vi "PrototypeV2_control.vi"() -> ()   [LabVIEW 2019]
uses:
  0f690846-c94a-4028-9fe1-d10e28cf598c.vi
  <vilib>/Instr/_visa.llb/VISA Configure Serial Port (Instr).vi
panel:
  out "elapsed time":dbl
  in  "SAS file":path
  in  "SAS VISA":refnum<visa-resource-name>
  out "CONV2":cluster{dbl, dbl, dbl}(graph)
  out "converter2 file":path
  out "controller file":path
  out "converter1 file":path
  in  "CONVERTER 2 PORT":refnum<visa-resource-name>="COM5"
  out "sync":bool
  in  "CONVERTER 1 PORT":refnum<visa-resource-name>="COM4"
  out "sync":bool
  out "CONV1":cluster{dbl, dbl, dbl}(graph)
  out "3.3V REG":cluster{dbl, dbl}(graph)
  out "5V REG":cluster{dbl, dbl}(graph)
  out "BUS":cluster{dbl, dbl, dbl}(graph)
  in  "project name":string
  in  "START":bool
  in  "CONTROLLER PORT":refnum<visa-resource-name>="COM3"
  out "sync":bool
  in  "STOP":bool
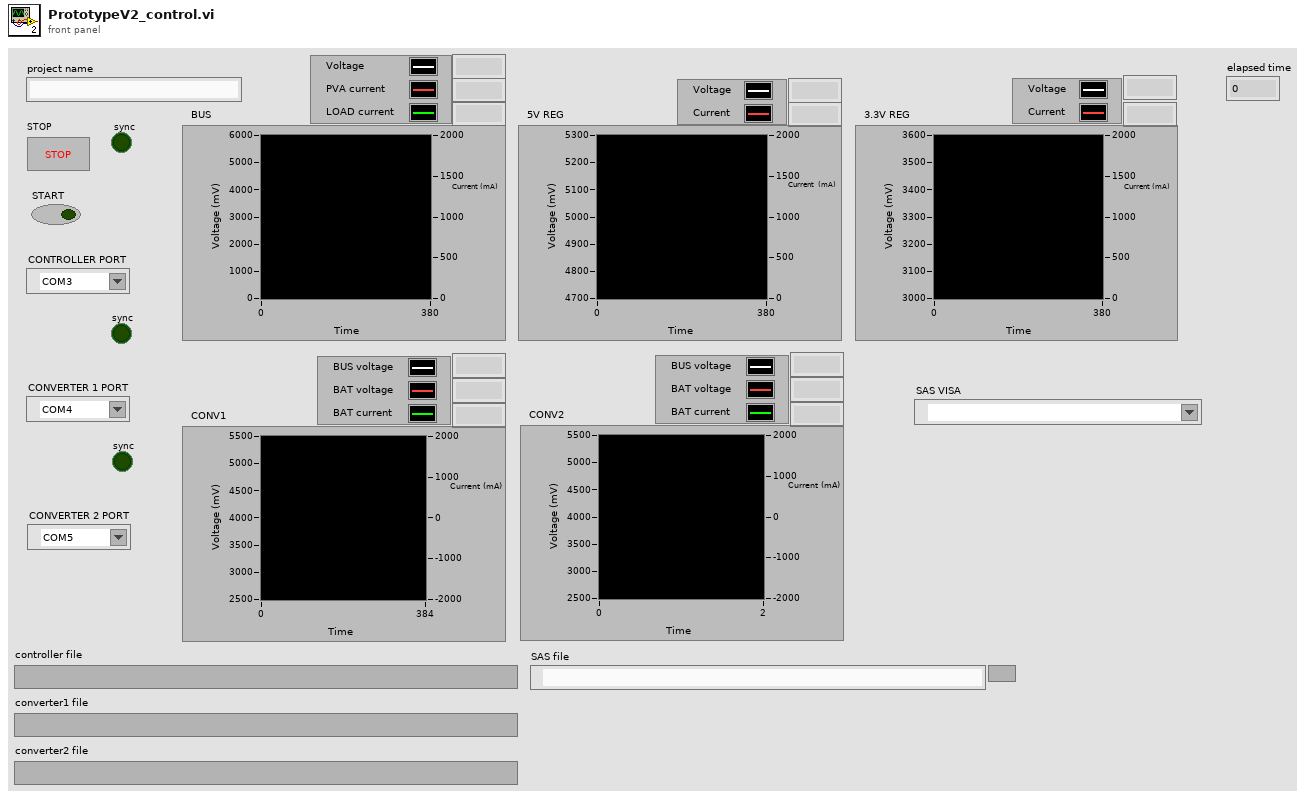
[diagram p1: front panel]
types:
  T1 = cluster{u16, u16, u16, u16, u16, u16, u16, u16, u16}
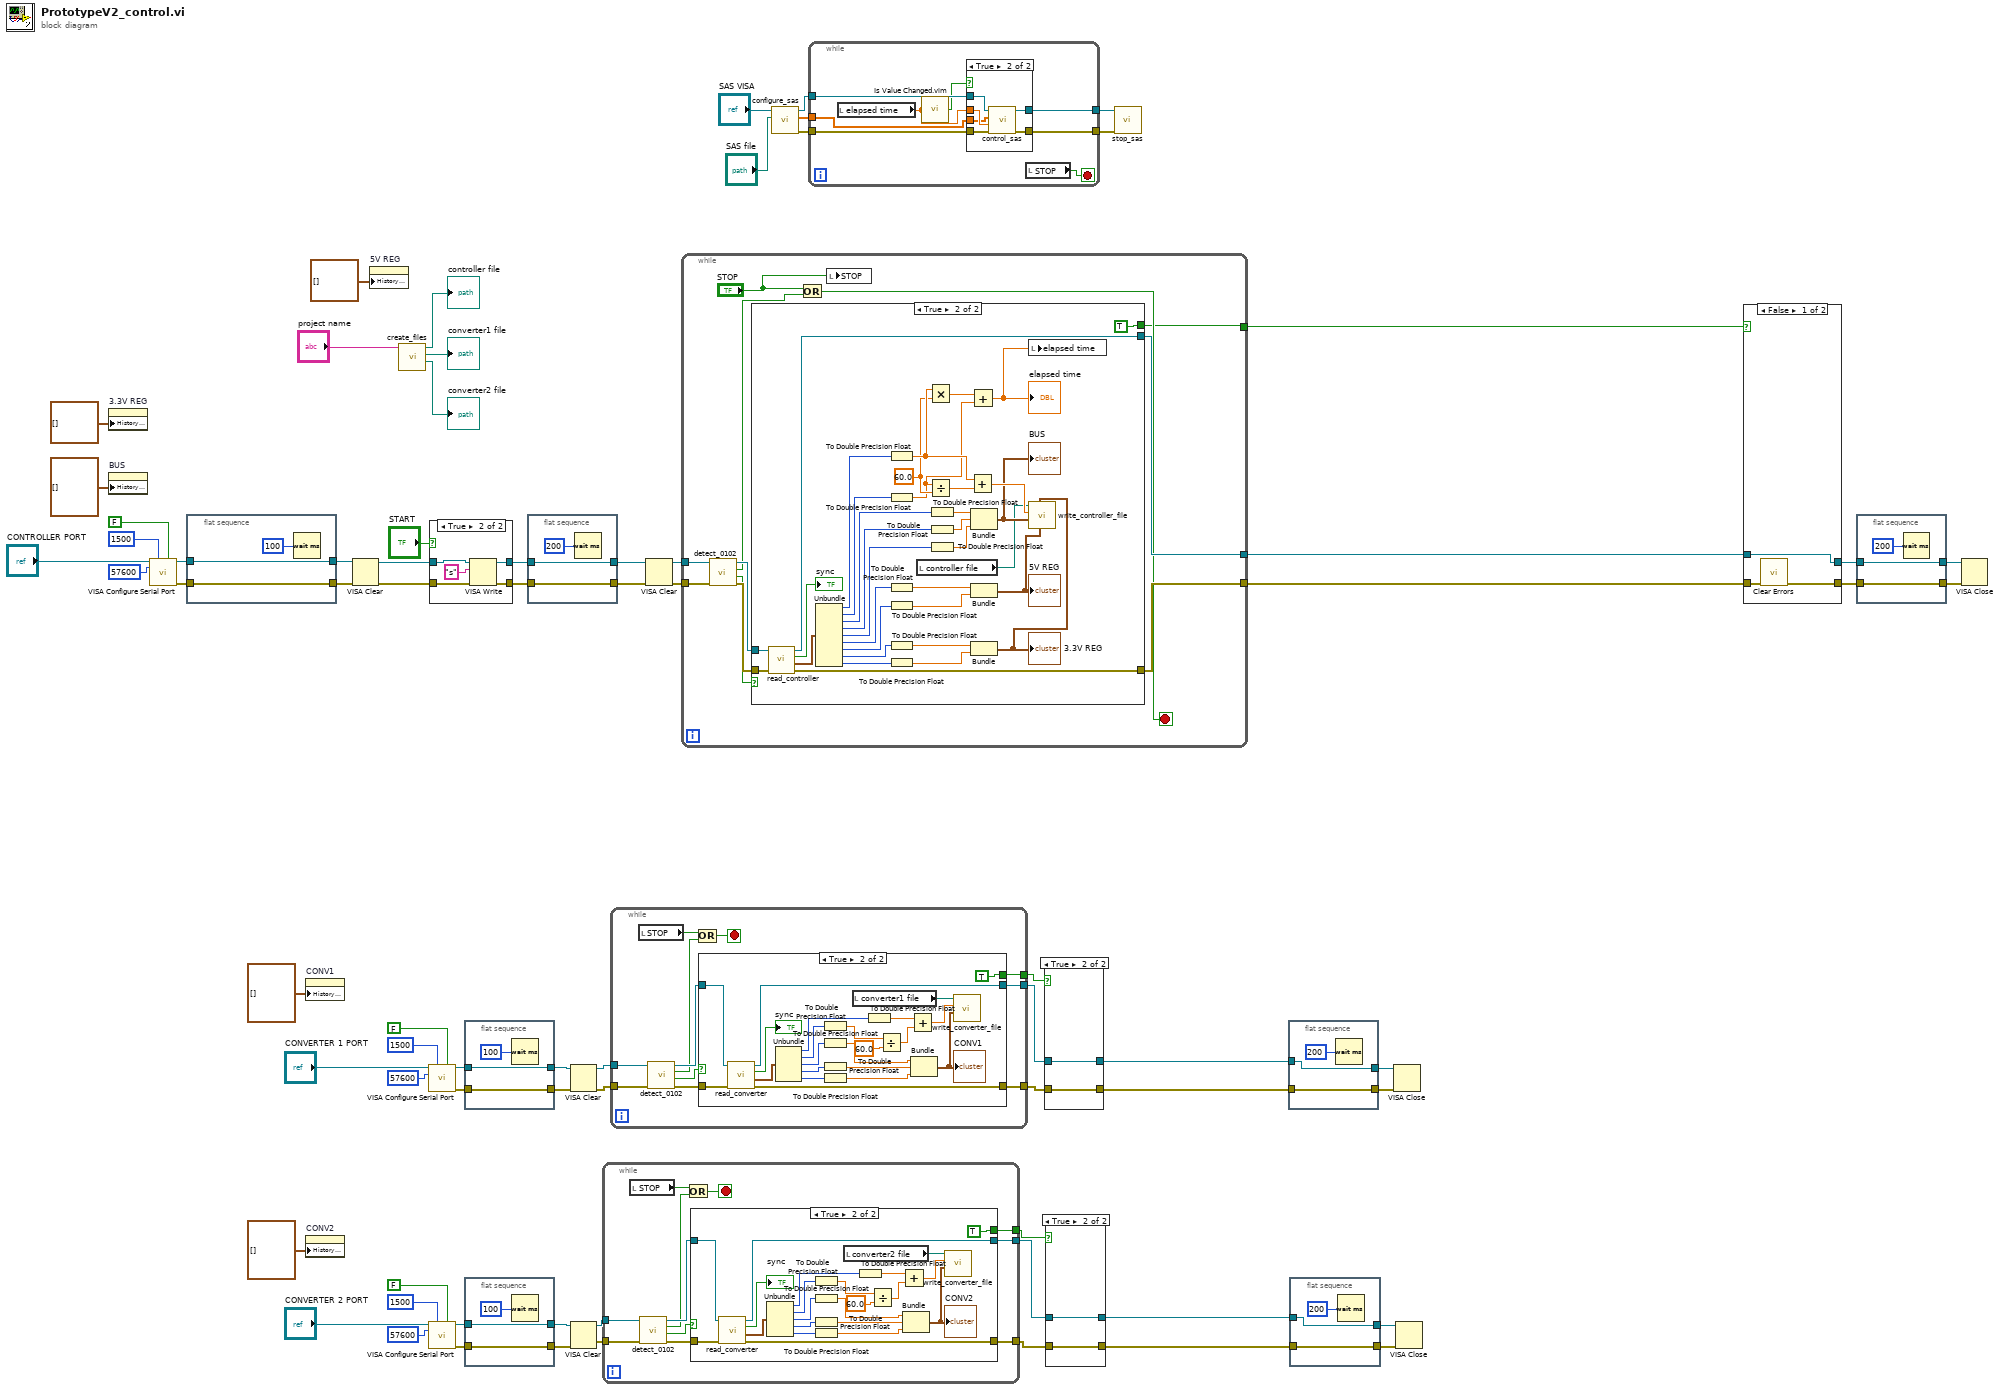
[diagram p0: block diagram]
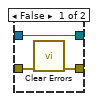
[diagram p3: hidden frame]
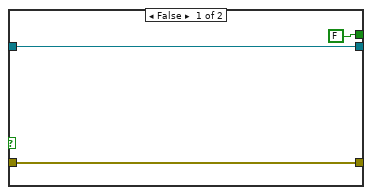
[diagram p4: hidden frame]
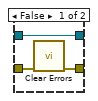
[diagram p5: hidden frame]
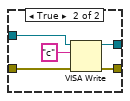
[diagram p6: hidden frame]
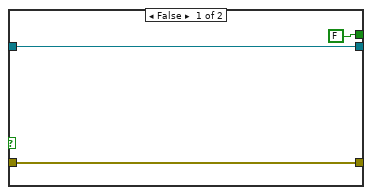
[diagram p7: hidden frame]
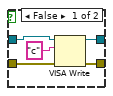
[diagram p8: hidden frame]
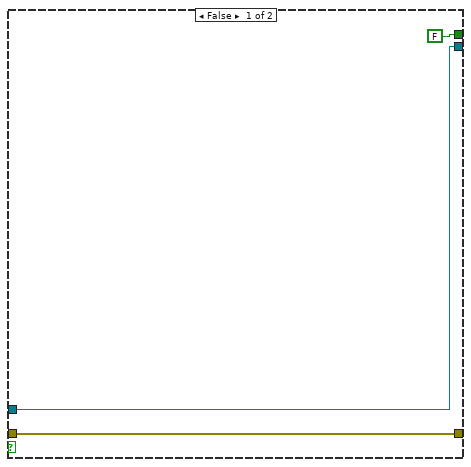
[diagram p9: hidden frame]
diagram:
  n1 = property on="3.3V REG" class="WFChart (strict)"("History Data"=cluster{dbl, dbl}[] []) -> ()  [unwired: 2 in, 2 out]
  n2 = property on="BUS" class="WFChart (strict)"("History Data"=cluster{dbl, dbl, dbl}[] []) -> ()  [unwired: 2 in, 2 out]
  n3 = call-poly "VISA Configure Serial Port"("VISA resource name"="CONTROLLER PORT", "timeout (10sec)"=u32 1500, "Enable Termination\nChar (T)"=FALSE ("Enable Termination\nChar (T)"), "baud rate (9600)"=u32 57600) -> ("VISA resource name out"=w71:refnum<visa-resource-name>, "error out"=w70:errorcluster)  [unwired: 10 in]
  n4 = flat-sequence {
    tunnel: w70 -> [w76]
    tunnel: [w76] -> w69
    tunnel: [w75] -> w68
    tunnel: w71 -> [w75]
    frame #0 {
      n5 = Wait (ms)(milliseconds to wait=u32 100) -> ()  [unwired: 1 out]
    }
  }
  n6 = property on="CONV1" class="WFChart (strict)"("History Data"=cluster{dbl, dbl, dbl}[] []) -> ()  [unwired: 2 in, 2 out]
  n7 = property on="CONV2" class="WFChart (strict)"("History Data"=cluster{dbl, dbl, dbl}[] []) -> ()  [unwired: 2 in, 2 out]
  n8 = VISA Clear(VISA resource name=w68, error in (no error)=w69) -> (VISA resource name out=w67:refnum<visa-resource-name>, error out=w66:errorcluster)
  n9 = property on="5V REG" class="WFChart (strict)"("History Data"=cluster{dbl, dbl}[] []) -> ()  [unwired: 2 in, 2 out]
  n10 = call "create_files.vi"("project name"="project name") -> ("converter2"=→"converter2 file":path, "converter1"=→"converter1 file":path, "controller"=→"controller file":path)  [unwired: 8 in]
  n11 = call-poly "VISA Configure Serial Port"("VISA resource name"="CONVERTER 1 PORT", "timeout (10sec)"=u32 1500, "Enable Termination\nChar (T)"=FALSE ("Enable Termination\nChar (T)"), "baud rate (9600)"=u32 57600) -> ("VISA resource name out"=w46:refnum<visa-resource-name>, "error out"=w45:errorcluster)  [unwired: 10 in]
  n12 = call-poly "VISA Configure Serial Port"("VISA resource name"="CONVERTER 2 PORT", "timeout (10sec)"=u32 1500, "Enable Termination\nChar (T)"=FALSE ("Enable Termination\nChar (T)"), "baud rate (9600)"=u32 57600) -> ("VISA resource name out"=w23:refnum<visa-resource-name>, "error out"=w22:errorcluster)  [unwired: 10 in]
  n13 = case shown="True" "START" {
    tunnel: w67 -> [w81 w87]
    tunnel: [w79 w86] -> w64
    tunnel: w66 -> [w80 w85]
    tunnel: [w78 w84] -> w63
    frame False {
      n14 = VISA Write(VISA resource name=w81, write buffer="c", error in (no error)=w80) -> (VISA resource name out=w79:refnum<visa-resource-name>, error out=w78:errorcluster)  [unwired: 1 out]
    }
    frame True {
      n15 = VISA Write(VISA resource name=w87, write buffer="s", error in (no error)=w85) -> (VISA resource name out=w86:refnum<visa-resource-name>, error out=w84:errorcluster)  [unwired: 1 out]
    }
  }
  n16 = flat-sequence {
    tunnel: w45 -> [w89]
    tunnel: [w89] -> w44
    tunnel: [w88] -> w43
    tunnel: w46 -> [w88]
    frame #0 {
      n17 = Wait (ms)(milliseconds to wait=u32 100) -> ()  [unwired: 1 out]
    }
  }
  n18 = flat-sequence {
    tunnel: w22 -> [w92]
    tunnel: [w92] -> w21
    tunnel: [w91] -> w20
    tunnel: w23 -> [w91]
    frame #0 {
      n19 = Wait (ms)(milliseconds to wait=u32 100) -> ()  [unwired: 1 out]
    }
  }
  n20 = flat-sequence {
    tunnel: w63 -> [w95]
    tunnel: [w95] -> w60
    tunnel: [w94] -> w62
    tunnel: w64 -> [w94]
    frame #0 {
      n21 = Wait (ms)(milliseconds to wait=u32 200) -> ()  [unwired: 1 out]
    }
  }
  n22 = VISA Clear(VISA resource name=w43, error in (no error)=w44) -> (VISA resource name out=w28:refnum<visa-resource-name>, error out=w27:errorcluster)
  n23 = VISA Clear(VISA resource name=w20, error in (no error)=w21) -> (VISA resource name out=w11:refnum<visa-resource-name>, error out=w10:errorcluster)
  n24 = while {
    tunnel: w10 -> [w102]
    tunnel: [w106] -> w13
    tunnel: [w107] -> w14
    tunnel: w11 -> [w103]
    tunnel: [w104] -> w12
    stop <- w105 stop-if-true
    n25 = local read "STOP"() -> (w97:bool)
    n26 = call "detect_0102.vi"("error in (no error)"=w102, "VISA Refnum in"=w103) -> ("error out"=w100:errorcluster, "RECEIVED"=w98:bool, "NOT RECEIVED"=w99:bool, "VISA Refnum out"=w101:refnum<visa-resource-name>)  [unwired: 6 in]
    n27 = Or(x=w97, y=w99) -> (x .or. y?=w105:bool)
    n28 = case shown="True" w98 {
      tunnel: w101 -> [w110 w119]
      tunnel: w100 -> [w109 w115]
      tunnel: [w110 w116] -> w107
      tunnel: [w109 w118] -> w106
      tunnel: [FALSE TRUE] -> w104
      frame False {
      }
      frame True {
        n29 = call "read_converter.vi"("error in (no error)"=w115, "VISA Refnum in"=w119) -> ("error out"=w118:errorcluster, "Types?"=w117:cluster{u16, u16, u16, u16, i16}, "sync"=→"sync":bool, "VISA Refnum out"=w116:refnum<visa-resource-name>)  [unwired: 6 in]
        n30 = Unbundle(w117) -> (w132:u16, w131:u16, w126:u16, w125:u16, w124:i16)
        n31 = To Double Precision Float(number=w131) -> (double precision float=w129:dbl)
        n32 = To Double Precision Float(number=w126) -> (double precision float=w123:dbl)
        n33 = To Double Precision Float(number=w125) -> (double precision float=w122:dbl)
        n34 = To Double Precision Float(number=w124) -> (double precision float=w121:dbl)
        n35 = local read "converter2 file"() -> (w111:path)
        n36 = To Double Precision Float(number=w132) -> (double precision float=w128:dbl)
        n37 = Divide(x=w129, y=60.0) -> (x/y=w127:dbl)
        n38 = Add(x=w128, y=w127) -> (x+y=w112:dbl)
        n39 = Bundle(w123, w122, w121) -> (w113:cluster{dbl, dbl, dbl})  [unwired: 1 in]
        "CONV2" <- w113
        n40 = call "write_converter_file.vi"("CONVERTER"=w113, "minutes"=w112, "converter file"=w111) -> ()  [unwired: 9 in]
      }
    }
  }
  n41 = while {
    tunnel: w27 -> [w138]
    tunnel: [w142] -> w34
    tunnel: [w143] -> w35
    tunnel: w28 -> [w139]
    tunnel: [w140] -> w33
    stop <- w141 stop-if-true
    n42 = local read "STOP"() -> (w133:bool)
    n43 = call "detect_0102.vi"("error in (no error)"=w138, "VISA Refnum in"=w139) -> ("error out"=w136:errorcluster, "RECEIVED"=w134:bool, "NOT RECEIVED"=w135:bool, "VISA Refnum out"=w137:refnum<visa-resource-name>)  [unwired: 6 in]
    n44 = Or(x=w133, y=w135) -> (x .or. y?=w141:bool)
    n45 = case shown="True" w134 {
      tunnel: w137 -> [w146 w155]
      tunnel: w136 -> [w145 w150]
      tunnel: [w146 w151] -> w143
      tunnel: [w145 w154] -> w142
      tunnel: [FALSE TRUE] -> w140
      frame False {
      }
      frame True {
        n46 = call "read_converter.vi"("error in (no error)"=w150, "VISA Refnum in"=w155) -> ("error out"=w154:errorcluster, "Types?"=w152:cluster{u16, u16, u16, u16, i16}, "sync"=→"sync":bool, "VISA Refnum out"=w151:refnum<visa-resource-name>)  [unwired: 6 in]
        n47 = Unbundle(w152) -> (w168:u16, w167:u16, w162:u16, w161:u16, w160:i16)
        n48 = To Double Precision Float(number=w167) -> (double precision float=w165:dbl)
        n49 = To Double Precision Float(number=w162) -> (double precision float=w159:dbl)
        n50 = To Double Precision Float(number=w161) -> (double precision float=w158:dbl)
        n51 = To Double Precision Float(number=w160) -> (double precision float=w157:dbl)
        n52 = local read "converter1 file"() -> (w148:path)
        n53 = To Double Precision Float(number=w168) -> (double precision float=w164:dbl)
        n54 = Divide(x=w165, y=60.0) -> (x/y=w163:dbl)
        n55 = Add(x=w164, y=w163) -> (x+y=w149:dbl)
        n56 = Bundle(w159, w158, w157) -> (w147:cluster{dbl, dbl, dbl})  [unwired: 1 in]
        "CONV1" <- w147
        n57 = call "write_converter_file.vi"("CONVERTER"=w147, "minutes"=w149, "converter file"=w148) -> ()  [unwired: 9 in]
      }
    }
  }
  n58 = VISA Clear(VISA resource name=w62, error in (no error)=w60) -> (VISA resource name out=w61:refnum<visa-resource-name>, error out=w59:errorcluster)
  n59 = while {
    tunnel: w59 -> [w177]
    tunnel: [w174] -> w57
    tunnel: [w175] -> w58
    tunnel: w61 -> [w176]
    tunnel: [w170] -> w41
    stop <- w173 stop-if-true
    n60 = call "detect_0102.vi"("error in (no error)"=w177, "VISA Refnum in"=w176) -> ("error out"=w178:errorcluster, "RECEIVED"=w171:bool, "NOT RECEIVED"=w172:bool, "VISA Refnum out"=w179:refnum<visa-resource-name>)  [unwired: 6 in]
    n61 = case shown="True" w171 {
      tunnel: w179 -> [w182 w216]
      tunnel: w178 -> [w181 w215]
      tunnel: [w182 w207] -> w175
      tunnel: [w181 w206] -> w174
      tunnel: [FALSE TRUE] -> w170
      frame False {
      }
      frame True {
        w186 = 60.0 ("y")
        n62 = call "read_controller.vi"("error in (no error)"=w215, "VISA Refnum in"=w216) -> ("error out"=w206:errorcluster, "Type?"=w214:T1, "sync"=→"sync":bool, "VISA Refnum out"=w207:refnum<visa-resource-name>)  [unwired: 6 in]
        n63 = Unbundle(w214) -> (w213:u16, w212:u16, w210:u16, w209:u16, w208:u16, w205:u16, w204:u16, w203:u16, w202:u16)
        n64 = To Double Precision Float(number=w213) -> (double precision float=w187:dbl)
        n65 = To Double Precision Float(number=w212) -> (double precision float=w184:dbl)
        n66 = To Double Precision Float(number=w205) -> (double precision float=w201:dbl)
        n67 = To Double Precision Float(number=w204) -> (double precision float=w200:dbl)
        n68 = To Double Precision Float(number=w203) -> (double precision float=w199:dbl)
        n69 = To Double Precision Float(number=w202) -> (double precision float=w198:dbl)
        n70 = local read "controller file"() -> (w190:path)
        n71 = Multiply(x=w187, y=w186) -> (x*y=w185:dbl)
        n72 = Divide(x=w184, y=w186) -> (x/y=w211:dbl)
        n73 = To Double Precision Float(number=w210) -> (double precision float=w194:dbl)
        n74 = To Double Precision Float(number=w209) -> (double precision float=w195:dbl)
        n75 = To Double Precision Float(number=w208) -> (double precision float=w196:dbl)
        n76 = Add(x=w187, y=w211) -> (x+y=w192:dbl)
        n77 = Add(x=w185, y=w184) -> (x+y=w183:dbl)
        "elapsed time" <- w183
        n78 = Bundle(w194, w195, w196) -> (w191:cluster{dbl, dbl, dbl})  [unwired: 1 in]
        "BUS" <- w191
        n79 = Bundle(w201, w200) -> (w189:cluster{dbl, dbl})  [unwired: 1 in]
        "5V REG" <- w189
        n80 = Bundle(w199, w198) -> (w188:cluster{dbl, dbl})  [unwired: 1 in]
        "3.3V REG" <- w188
        n81 = local write "elapsed time"(w183) -> ()
        n82 = call "write_controller_file.vi"("5V reg"=w189, "3.3V reg"=w188, "BUS"=w191, "minutes"=w192, "controller file"=w190) -> ()  [unwired: 7 in]
      }
    }
    n83 = Or(x="STOP", y=w172) -> (x .or. y?=w173:bool)
    n84 = local write "STOP"("STOP") -> ()
  }
  n85 = call "configure_sas.vi"("SAS file"="SAS file", "VISA Refnum in"="SAS VISA") -> ("error out"=w4:errorcluster, "all rows"=w3:dbl[], "VISA Refnum out"=w5:refnum<visa-resource-name>)  [unwired: 5 in]
  n86 = while {
    tunnel: w5 -> [w224]
    tunnel: w4 -> [w223]
    tunnel: w3 -> [w222]
    tunnel: [w218] -> w2
    tunnel: [w217] -> w1
    stop <- w219 stop-if-true
    n87 = local read "elapsed time"() -> (w221:dbl)
    n88 = call "Is Value Changed.vim"("value"=w221) -> ("changed or first call?"=w220:bool)
    n89 = case shown="True" w220 {
      tunnel: w224 -> [w226 w232]
      tunnel: w223 -> [w225 w231]
      tunnel: w221 -> [_ w230]
      tunnel: w222 -> [_ w229]
      tunnel: [w226 w228] -> w218
      tunnel: [w225 w227] -> w217
      frame False {
      }
      frame True {
        n90 = call "control_sas.vi"("error in (no error)"=w231, "Numeric"=w230, "all rows"=w229, "VISA Refnum in"=w232) -> ("error out"=w227:errorcluster, "VISA Refnum out"=w228:refnum<visa-resource-name>)  [unwired: 6 in]
      }
    }
    n91 = local read "STOP"() -> (w219:bool)
  }
  n92 = case shown="True" w33 {
    tunnel: w35 -> [w235 w237]
    tunnel: w34 -> [w234 w236]
    tunnel: [w235 w237] -> w39
    tunnel: [w233 w236] -> w38
    frame False {
      n93 = call <vilib>:"Clear Errors.vi"("error in (no error)"=w234) -> ("error out"=w233:errorcluster)  [unwired: 5 in, 1 out]
    }
    frame True {
    }
  }
  n94 = case shown="True" w12 {
    tunnel: w14 -> [w240 w242]
    tunnel: w13 -> [w239 w241]
    tunnel: [w240 w242] -> w18
    tunnel: [w238 w241] -> w17
    frame False {
      n95 = call <vilib>:"Clear Errors.vi"("error in (no error)"=w239) -> ("error out"=w238:errorcluster)  [unwired: 5 in, 1 out]
    }
    frame True {
    }
  }
  n96 = call "stop_sas.vi"("error in (no error)"=w1, "VISA Refnum in"=w2) -> ()  [unwired: 10 in]
  n97 = flat-sequence {
    tunnel: w38 -> [w244]
    tunnel: [w244] -> w37
    tunnel: [w243] -> w36
    tunnel: w39 -> [w243]
    frame #0 {
      n98 = Wait (ms)(milliseconds to wait=u32 200) -> ()  [unwired: 1 out]
    }
  }
  n99 = flat-sequence {
    tunnel: w17 -> [w247]
    tunnel: [w247] -> w16
    tunnel: [w246] -> w15
    tunnel: w18 -> [w246]
    frame #0 {
      n100 = Wait (ms)(milliseconds to wait=u32 200) -> ()  [unwired: 1 out]
    }
  }
  n101 = VISA Close(VISA resource name=w36, error in (no error)=w37) -> ()  [unwired: 1 out]
  n102 = VISA Close(VISA resource name=w15, error in (no error)=w16) -> ()  [unwired: 1 out]
  n103 = case shown="False" w41 {
    tunnel: w58 -> [w251 w255]
    tunnel: w57 -> [w250 w254]
    tunnel: [w251 w253] -> w56
    tunnel: [w249 w252] -> w55
    frame False {
      n104 = call <vilib>:"Clear Errors.vi"("error in (no error)"=w250) -> ("error out"=w249:errorcluster)  [unwired: 5 in, 1 out]
    }
    frame True {
      n105 = VISA Write(VISA resource name=w255, write buffer="c", error in (no error)=w254) -> (VISA resource name out=w253:refnum<visa-resource-name>, error out=w252:errorcluster)  [unwired: 1 out]
    }
  }
  n106 = flat-sequence {
    tunnel: w55 -> [w258]
    tunnel: [w258] -> w54
    tunnel: [w257] -> w53
    tunnel: w56 -> [w257]
    frame #0 {
      n107 = Wait (ms)(milliseconds to wait=u32 200) -> ()  [unwired: 1 out]
    }
  }
  n108 = VISA Close(VISA resource name=w53, error in (no error)=w54) -> ()  [unwired: 1 out]
